vi "set_CLUT.vi"(11 "file path":path=path "C:/Users/Thor/Documents/MM_LabView/CLUT_594.csv") -> (0 "error out":errorcluster, 1 "heds error":string)   [LabVIEW 2025]
uses:
  <vilib>/Utility/file.llb/Read Delimited Spreadsheet (I64).vi
  Desktop/matlab_controlfunc/holoeye_slmconfigsdk.dll
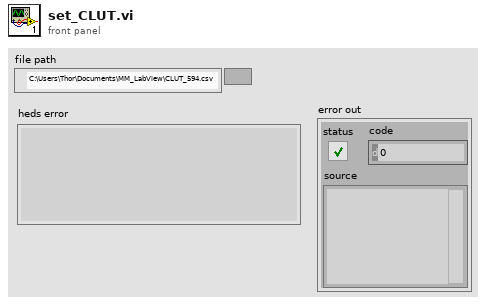
[diagram p1: front panel]
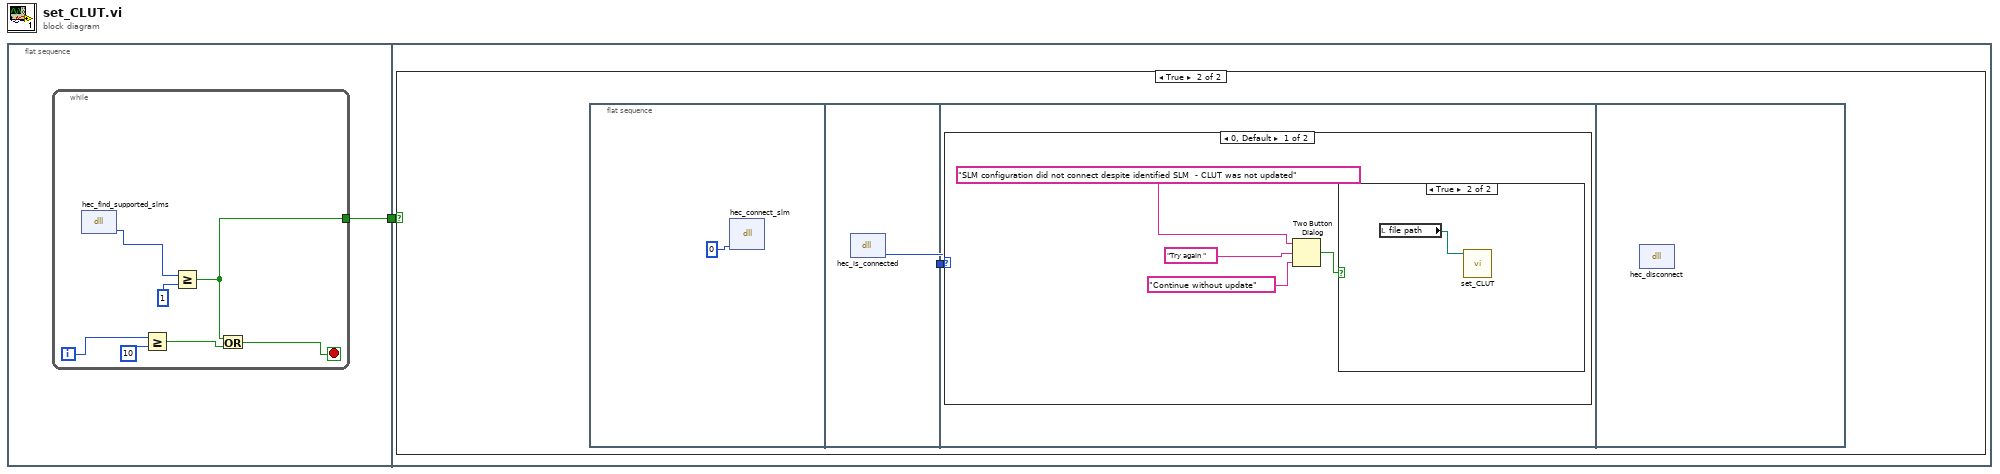
[diagram p0: block diagram]
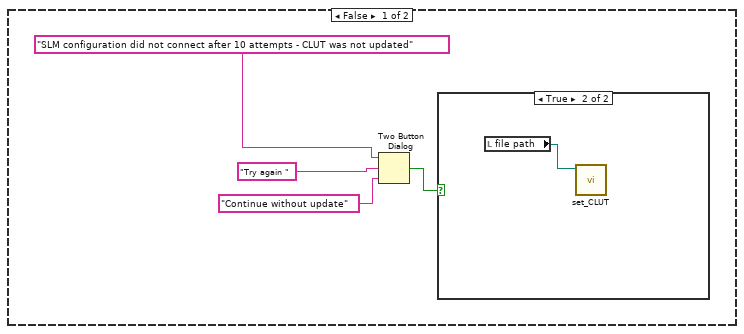
[diagram p2: hidden frame]
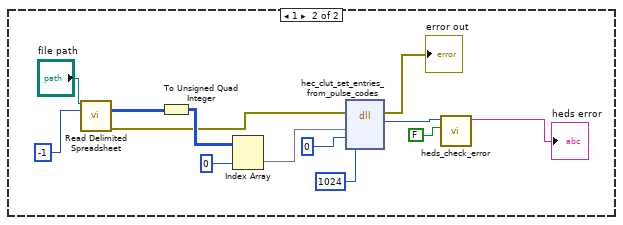
[diagram p5: hidden frame]
diagram:
  n1 = flat-sequence {
    tunnel: [w2] -> w1
    tunnel: w1 -> [w10]
    frame #0 {
      n2 = while {
        tunnel: [w4] -> w2
        i -> [w3]
        stop <- w7 stop-if-true
        n3 = dll-call lib="C:/Users/Thor/Desktop/matlab_controlfunc/holoeye_slmconfigsdk.dll" fn="hec_find_supported_slms"() -> ("number"=w6:i32)  [unwired: 3 in, 2 out]
        n4 = Greater Or Equal?(x=w3, y=10) -> (x >= y?=w8:bool)
        n5 = Greater Or Equal?(x=w6, y=1) -> (x >= y?=w4:bool)
        n6 = Or(x=w4, y=w8) -> (x .or. y?=w7:bool)
      }
    }
    frame #1 {
      n7 = case shown="True" w10 {
        frame False {
          n8 = Two Button Dialog(message="SLM configuration did not connect after 10 attempts - CLUT was not updated", 1:"Continue without update" ("F button name (\"Cancel\")"), 2:"Try again " ("T button name (\"OK\")")) -> (T button?=w11:bool)
          n9 = case shown="True" w11 {
            frame False {
            }
            frame True {
              n10 = local read "file path"() -> (w15:path)
              n11 = call "set_CLUT.vi"("file path"=w15) -> ()  [unwired: 9 in, 2 out]
            }
          }
        }
        frame True {
          n12 = flat-sequence {
            tunnel: [w18] -> w16
            tunnel: w16 -> [w19]
            frame #0 {
              n13 = dll-call lib="C:/Users/Thor/Desktop/matlab_controlfunc/holoeye_slmconfigsdk.dll" fn="hec_connect_slm"("slmNumber"=u32 0) -> ()  [unwired: 5 in, 2 out]
            }
            frame #1 {
              n14 = dll-call lib="C:/Users/Thor/Desktop/matlab_controlfunc/holoeye_slmconfigsdk.dll" fn="hec_is_connected"() -> ("isconnected"=w18:i32)  [unwired: 3 in, 2 out]
            }
            frame #2 {
              n15 = case shown="0, Default" w19 {
                frame 0, Default {
                  n16 = Two Button Dialog(message="SLM configuration did not connect despite identified SLM  - CLUT was not updated", 1:"Continue without update" ("F button name (\"Cancel\")"), 2:"Try again " ("T button name (\"OK\")")) -> (T button?=w20:bool)
                  n17 = case shown="True" w20 {
                    frame False {
                    }
                    frame True {
                      n18 = local read "file path"() -> (w24:path)
                      n19 = call "set_CLUT.vi"("file path"=w24) -> ()  [unwired: 9 in, 2 out]
                    }
                  }
                }
                frame 1 {
                  n20 = call-poly <vilib>:"Read Delimited Spreadsheet.vi"("file path (dialog if empty)"="file path", "number of rows (all:-1)"=-1) -> ("all rows"=w35:i64[][], "error out"=w31:errorcluster)  [unwired: 8 in, 4 out]
                  n21 = To Unsigned Quad Integer(1:w35) -> (0:w36:u64[][])
                  n22 = Index Array(array=w36, index (col)=0) -> (element=w37:u64[])  [unwired: 1 in]
                  n23 = dll-call lib="C:/Users/Thor/Desktop/matlab_controlfunc/holoeye_slmconfigsdk.dll" fn="hec_clut_set_entries_from_pulse_codes"(error in=w31, "clut"=w37, "HOLOEYE_DEFARG0"=0, "HOLOEYE_DEFARGneg1"=1024) -> (error out=→"error out":errorcluster, "error message"=w34:i32)  [unwired: 5 in, 1 out]
                  n24 = call <userlib>:"heds_check_error.vi"("Show Error Dialog"=FALSE, "error code"=w34) -> ("heds error string"=→"heds error":string)  [unwired: 8 in, 1 out]
                }
              }
            }
            frame #3 {
              n25 = dll-call lib="C:/Users/Thor/Desktop/matlab_controlfunc/holoeye_slmconfigsdk.dll" fn="hec_disconnect"() -> ()  [unwired: 4 in, 2 out]
            }
          }
        }
      }
    }
  }
